vi "P116x1ch_ZeroWriteAuto.vi"(8 "error in (no error)":errorcluster, 11 "Comunicaciones":T1={"Eurothe"="ASRL6::INSTR", "Eurot"=FALSE}) -> (0 "error out":errorcluster, 1 "RateSP(C/min) 2":T2, 2 "NuevoSP(C) 2":T2, 9 "Rate(C/min)":T2, 10 "SP(C)":T2)   [LabVIEW 2017]
uses:
  1xP116.ctl
  Controles/P2024 COMMS.ctl
  Eurotherm_Hardware_Module Control.ctl
  P2024 Eurotherm GLOBALES.vi
panel:
  out "PV":T2
  out "WorkingSP":T2
  out "TargetSP":T2
  in  "Cancel":bool
  in  "Write":bool
  out "Enable(T)":bool=TRUE
  out "VISA Promux":refnum<visa-resource-name>
  in  "Delay Time (s)":dbl=0.1
  # "Apagando Eurotherm"
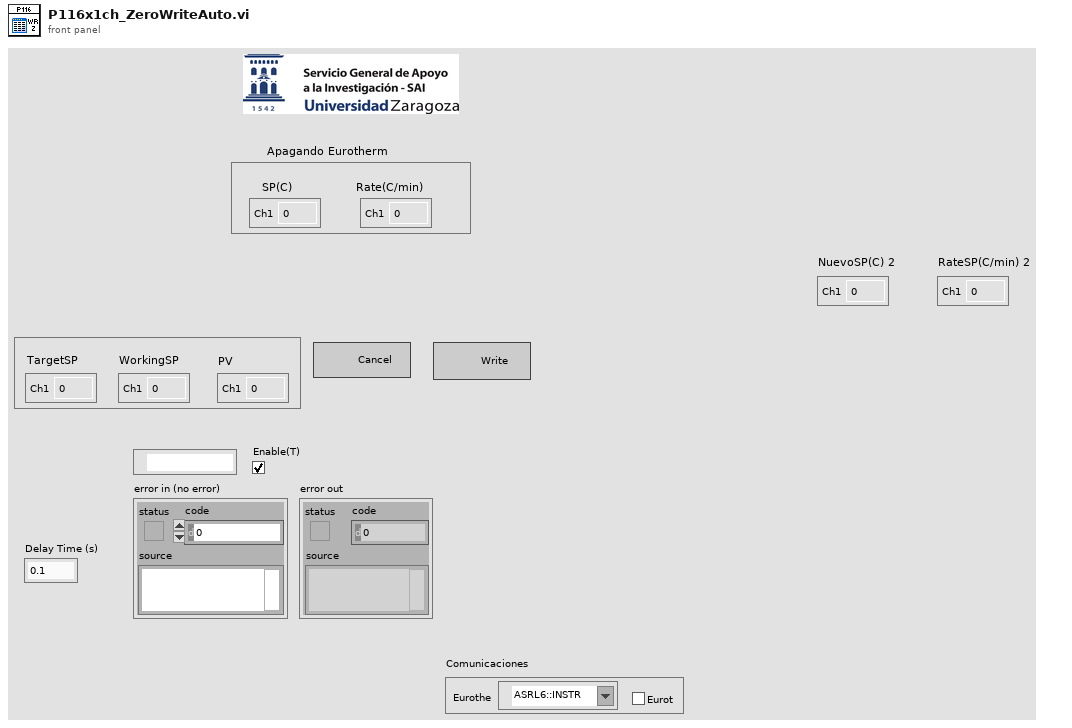
[diagram p1: front panel]
types:
  T1 = typedef "P2024 COMMS.ctl" = cluster{"Eurothe":refnum<visa-resource-name>, "Eurot":bool}
  T2 = typedef "1xP116.ctl" = cluster{"Ch1":dbl}
  T3 = cluster{"TargetSP":T2, "WorkingSP":T2, "Temperatura":T2, "Error":bool, "Date":string, "Delay(s)":dbl, "RateSP":T2, "Potencia":T2}
  T4 = typedef "Eurotherm_Hardware_Module Control.ctl" = enum16{"Initialize", "Write SP", "Read SP+PV", "Write Rate", "Set P", "Set I", "Set D", "Shutdown"}
  T5 = enum16{"Add 1", "Add 2", "Add 10", "Add 11", "Add 12", "Add 13"}[]
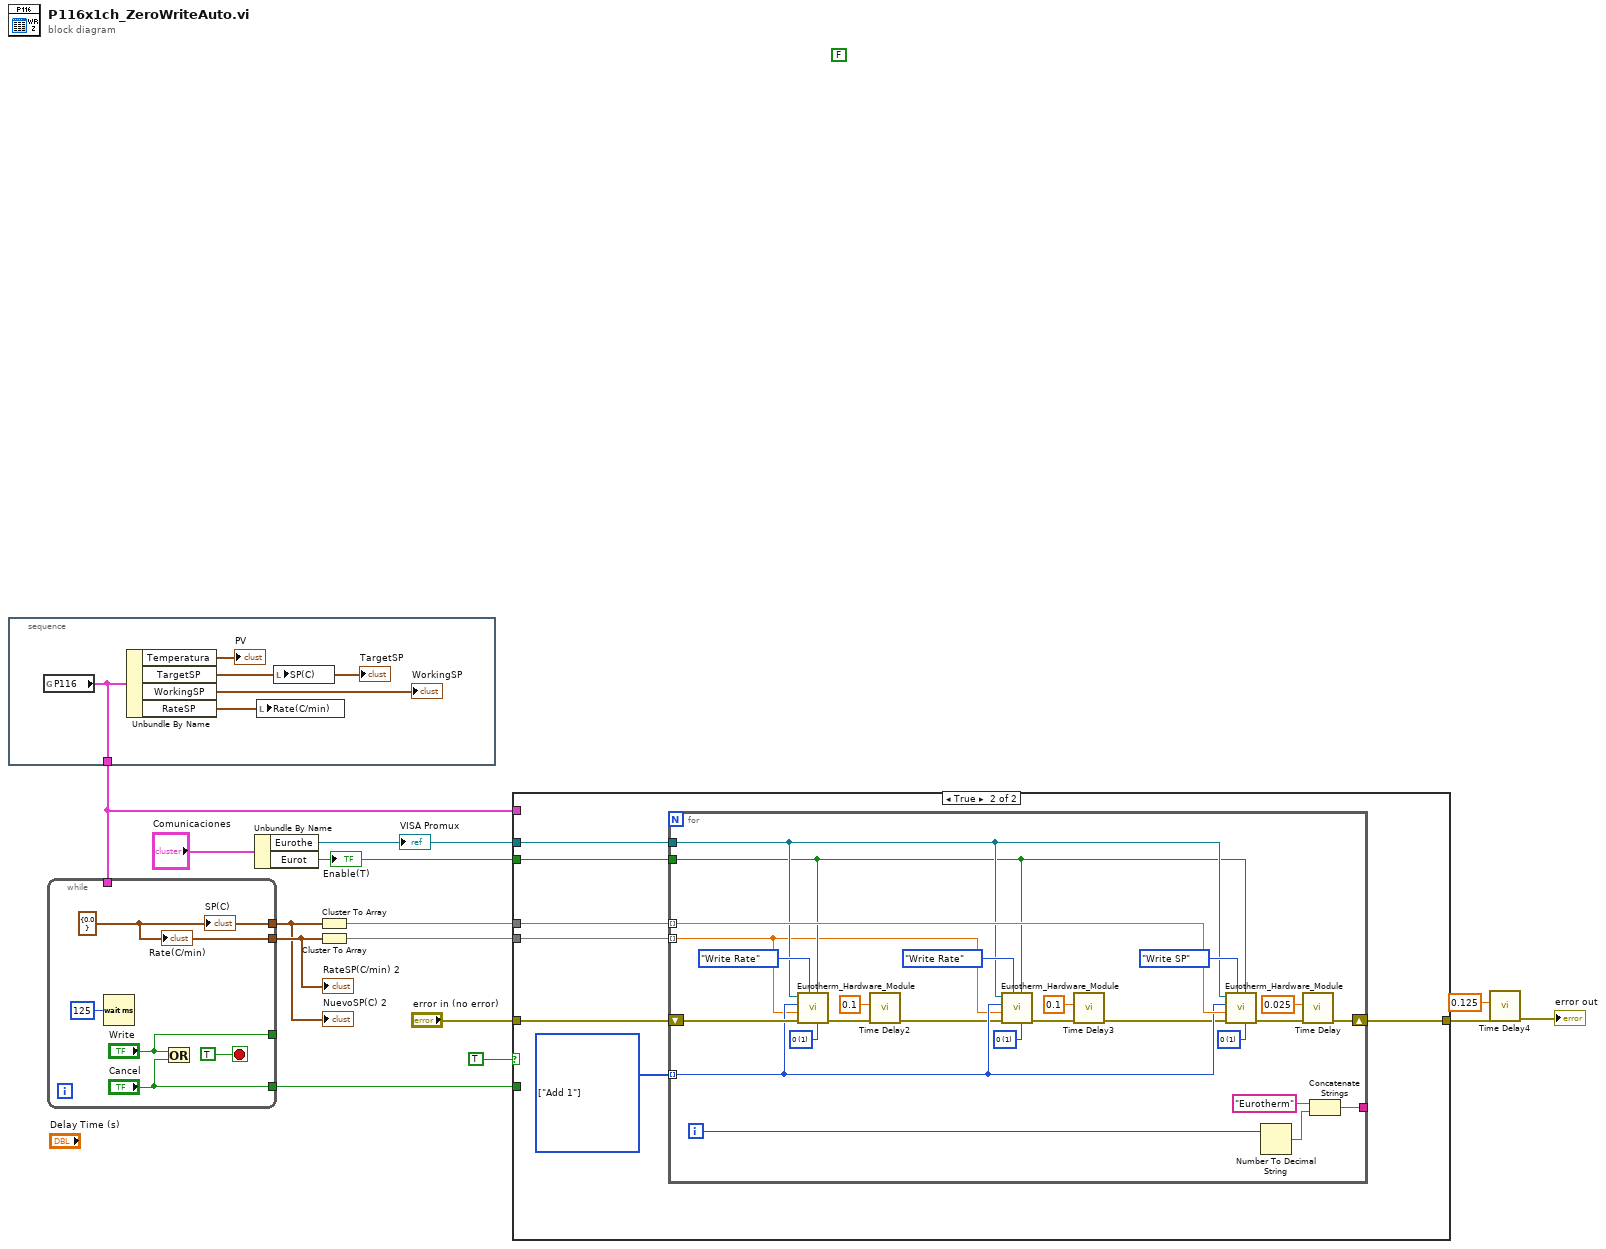
[diagram p0: block diagram]
diagram:
  (unwired) FALSE
  n1 = stacked-sequence {
    tunnel: [w16] -> w8
    frame #0 {
      n2 = global read "P2024 Eurotherm GLOBALES.vi" "P116"() -> (w16:T3)
      n3 = Unbundle By Name(w16) -> ("Temperatura"=→"PV":T2, "TargetSP"=w17:T2, "WorkingSP"=→"WorkingSP":T2, "RateSP"=w15:T2)
      "TargetSP" <- w17
      n4 = local write "Rate(C/min)"(w15) -> ()
      n5 = local write "SP(C)"(w17) -> ()
    }
  }
  n6 = while {
    tunnel: ["Cancel"] -> w13
    tunnel: [w21] -> w6
    tunnel: [w21] -> w7
    tunnel: ["Write"] -> _
    tunnel: w8 -> [_]
    stop <- TRUE stop-if-true
    w21 = T2 {"Ch1"=0.0} ("NuevoSP")
    n7 = Wait (ms)(milliseconds to wait=u32 125) -> ()  [unwired: 1 out]
    n8 = Or(x="Write", y="Cancel") -> ()  [unwired: 1 out]
    "Rate(C/min)" <- w21
    "SP(C)" <- w21
  }
  "NuevoSP(C) 2" <- w6
  "RateSP(C/min) 2" <- w7
  n9 = Unbundle By Name("Comunicaciones") -> ("Eurothe"=w9:refnum<visa-resource-name>, "Eurot"=w14:bool)
  "Enable(T)" <- w14
  "VISA Promux" <- w9
  n10 = Cluster To Array(cluster=w6) -> (array=w11:dbl[])
  n11 = Cluster To Array(cluster=w7) -> (array=w10:dbl[])
  n12 = case shown="True" TRUE {
    tunnel: w14 -> [_ w31]
    tunnel: w13 -> [_ _]
    tunnel: "error in (no error)" -> [w25 w30]
    tunnel: w11 -> [_ w28]
    tunnel: w10 -> [_ w29]
    tunnel: w9 -> [_ w32]
    tunnel: w8 -> [_ _]
    tunnel: [w25 w26] -> w3
    frame False {
    }
    frame True {
      w27 = T5 [enum."Add 1"] items=["Add 1", "Add 2", "Add 10", "Add 11", "Add 12", "Add 13"]
      n13 = for {
        tunnel: w27 -> [w38] mode=indexing
        shift-right: [w48] -> w26
        shift-left: w30 -> [w52]
        tunnel: [w55] -> _
        tunnel: w28 -> [w50] mode=indexing
        tunnel: w29 -> [w33] mode=indexing
        tunnel: w32 -> [w35]
        tunnel: w31 -> [w34]
        i -> [w47]
        w40 = u16 1 items=["0"=1, "1"=10, "2"=100] ("Decimales")
        w46 = u16 1 items=["0"=1, "1"=10, "2"=100] ("Decimales")
        w45 = u16 1 items=["0"=1, "1"=10, "2"=100] ("Decimales")
        n14 = call "Eurotherm_Hardware_Module.vi"("Decimales"=w46, "Eurotherm (T:Enable)"=w34, "Command"=Eurotherm_Hardware_Module_Control."Write Rate", "error in (no error)"=w52, "Value"=w33, "Address"=w38, "VISA resource name"=w35) -> ("error out"=w44:errorcluster)  [unwired: 2 in, 2 out]
        n15 = call "Time Delay2"("error in (no error)"=w44, "Delay Time (s)"=0.1) -> ("error out"=w37:errorcluster)  [unwired: 9 in]
        n16 = call "Eurotherm_Hardware_Module.vi"("Decimales"=w40, "Eurotherm (T:Enable)"=w34, "Command"=Eurotherm_Hardware_Module_Control."Write Rate", "error in (no error)"=w37, "Value"=w33, "Address"=w38, "VISA resource name"=w35) -> ("error out"=w41:errorcluster)  [unwired: 2 in, 2 out]
        n17 = call "Time Delay3"("error in (no error)"=w41, "Delay Time (s)"=0.1) -> ("error out"=w36:errorcluster)  [unwired: 9 in]
        n18 = call "Eurotherm_Hardware_Module.vi"("Decimales"=w45, "Eurotherm (T:Enable)"=w34, "Command"=Eurotherm_Hardware_Module_Control."Write SP", "error in (no error)"=w36, "Value"=w50, "Address"=w38, "VISA resource name"=w35) -> ("error out"=w49:errorcluster)  [unwired: 2 in, 2 out]
        n19 = Number To Decimal String(number=w47) -> (decimal integer string=w56:string)  [unwired: 1 in]
        n20 = call "Time Delay"("error in (no error)"=w49, "Delay Time (s)"=0.025) -> ("error out"=w48:errorcluster)  [unwired: 9 in]
        n21 = Concatenate Strings("Eurotherm" ("error source (\" \")"), w56) -> (w55:string)
      }
    }
  }
  n22 = call "Time Delay4"("error in (no error)"=w3, "Delay Time (s)"=0.125) -> ("error out"=→"error out":errorcluster)  [unwired: 9 in]
